vi "Initialize DAQ Instruments.vi"(8 "error in (no error)":errorcluster, 11 "DAQ":refnum<class "DAQ.lvclass">) -> (0 "error out":errorcluster, 3 "DAQ":refnum<class "DAQ.lvclass">)   [LabVIEW 2022 SP3, in "DAQ.lvclass"]
doc: "Developed by Kevin Thompson\nkevin@thompsonengineering.net\n\nCopyright 2018-2020\nThompson Engineering, LLC"
uses:
  DAQ.lvclass
  DAQ.lvclass/DAQ.ctl
  Accessors/Get DAQ Settings.vi
  Accessors/Set DI TaskNames.vi
  Accessors/Set AI TaskNames.vi
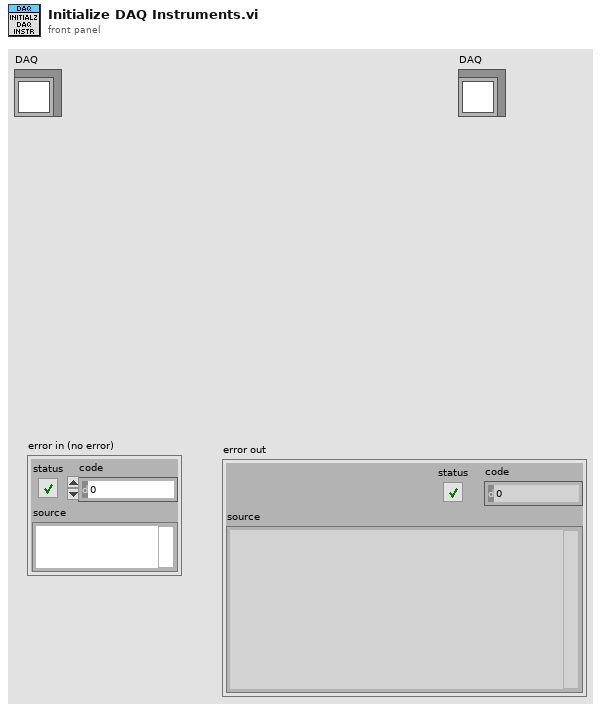
[diagram p1: front panel]
types:
  T1 = typedef "DAQ.lvclass/TD DAQ Settings--cluster.ctl" = cluster{"Simulate DAQ":bool, "DI Settings":T2[], "AI Settings":T3[], "Relay IONames":string[], "AO IONames":string[], "AO NChan SingleTask":bool}
  T2 = typedef "DAQ.lvclass/TD DI Instrument Settings--cluster.ctl" = cluster{"Disable":bool, "DI TaskName":string, "DI RefreshIntv":i32}
  T3 = typedef "DAQ.lvclass/TD AI Instrument Settings--cluster.ctl" = cluster{"Disable":bool, "AI TaskName":string, "AI InstSettings":T4, "SimAI Ranges":T5}
  T4 = typedef "DAQ.lvclass/TD AI InstSettings--cluster.ctl" = cluster{"DaqRate":dbl, "NumSamples":i32}
  T5 = typedef "DAQ.lvclass/TD SimAI Ranges--cluster.ctl" = cluster{"lo":dbl, "hi":dbl}
  T6 = typedef "TD Pathnames--cluster.ctl" = cluster{"RunTimeSys?":bool, "AppFolder":path, "ExecutablePath":path, "ConfigFolder":path, "DataLogFolder":path, "SystemLogFolder":path, "SeqFolder":path, "MainStartupPathname":path, "MainUIPathname":path, "SystemEventsFile":path, "SeqEventsFile":path, "Config SettingsFile":path, "DAQ IOConfigFile":path, "SystemSimulation":bool, "DLPUIConfigFile":path}
  T7 = typedef "TD Dynamic CVT DVR--ref.ctl" = refnum<data-value>
  T8 = typedef "DAQ.lvclass/TD IO Node Definition--cluster.ctl" = cluster{"DI Config":T9, "DO Config":T12, "AI Config":T14, "AO Config":T20}
  T9 = typedef "DAQ.lvclass/TD DI Config--cluster.ctl" = cluster{"DI Tasks":T10[]}
  T10 = typedef "DAQ.lvclass/TD DI Task--cluster.ctl" = cluster{"DI TaskName":string, "DI Channels":T11[]}
  T11 = typedef "DAQ.lvclass/TD DI Channel--cluster.ctl" = cluster{"DevName":string, "IOName":string, "IOPath":string, "SchemName":string, "logic":enum16{"Lo", "Hi"}, "Index":i32}
  T12 = typedef "DAQ.lvclass/TD DO Config--cluster.ctl" = cluster{"DO Channels":T13[]}
  T13 = typedef "DAQ.lvclass/TD DO Channel--cluster.ctl" = cluster{"DevName":string, "IOName":string, "IOPath":string, "SchemName":string, "logic":enum16{"Lo", "Hi"}, "DAQmx Task":refnum<k21>}
  T14 = typedef "DAQ.lvclass/TD AI Config--cluster.ctl" = cluster{"AI Tasks":T15[]}
  T15 = typedef "DAQ.lvclass/TD AI Task--cluster.ctl" = cluster{"AI TaskName":string, "AI Channels":T16[]}
  T16 = typedef "DAQ.lvclass/TD AI Channel--cluster.ctl" = cluster{"DevName":string, "IOName":string, "IOPath":string, "SchemName":string, "MinValue":dbl, "MaxValue":dbl, "Terminal Configuration":i32, "Index":i32, "Conversion":T17, "AIType":T18, "Force Bridge":T19}
  T17 = typedef "DAQ.lvclass/TD DataValueConversion--cluster.ctl" = cluster{"MaxSignal":dbl, "MinSignal":dbl, "MaxEngUnit":dbl, "MinEngUnit":dbl, "ScaleOffset":dbl, "negate":bool}
  T18 = typedef "DAQ.lvclass/TD AI DAQ Type--enum.ctl" = enum16{"Voltage", "Current", "Strain Gage", "Force Bridge"}
  T19 = typedef "DAQ.lvclass/TD AI Force Bridge--cluster.ctl" = cluster{"bridge information":cluster{"bridge configuration":i32, "voltage excitation source":i32, "voltage excitation value":dbl, "nominal bridge resistance":dbl}, "scaling information":cluster{"first electrical value":dbl, "second electrical value":dbl, "electrical units":i32, "first physical value":dbl, "second physical value":dbl, "physical units":i32}}
  T20 = typedef "DAQ.lvclass/TD AO Config--cluster.ctl" = cluster{"AO Channels":T21[]}
  T21 = typedef "DAQ.lvclass/TD AO Channel--cluster.ctl" = cluster{"DevName":string, "IOName":string, "IOPath":string, "SchemName":string, "Vmin":dbl, "Vmax":dbl, "Conversion":T17, "DAQmx Task":refnum<k21>}
  T22 = typedef "DAQ.lvclass/offsets cluster.ctl" = cluster{"Offset IONames":string[], "Offset Value":dbl[]}
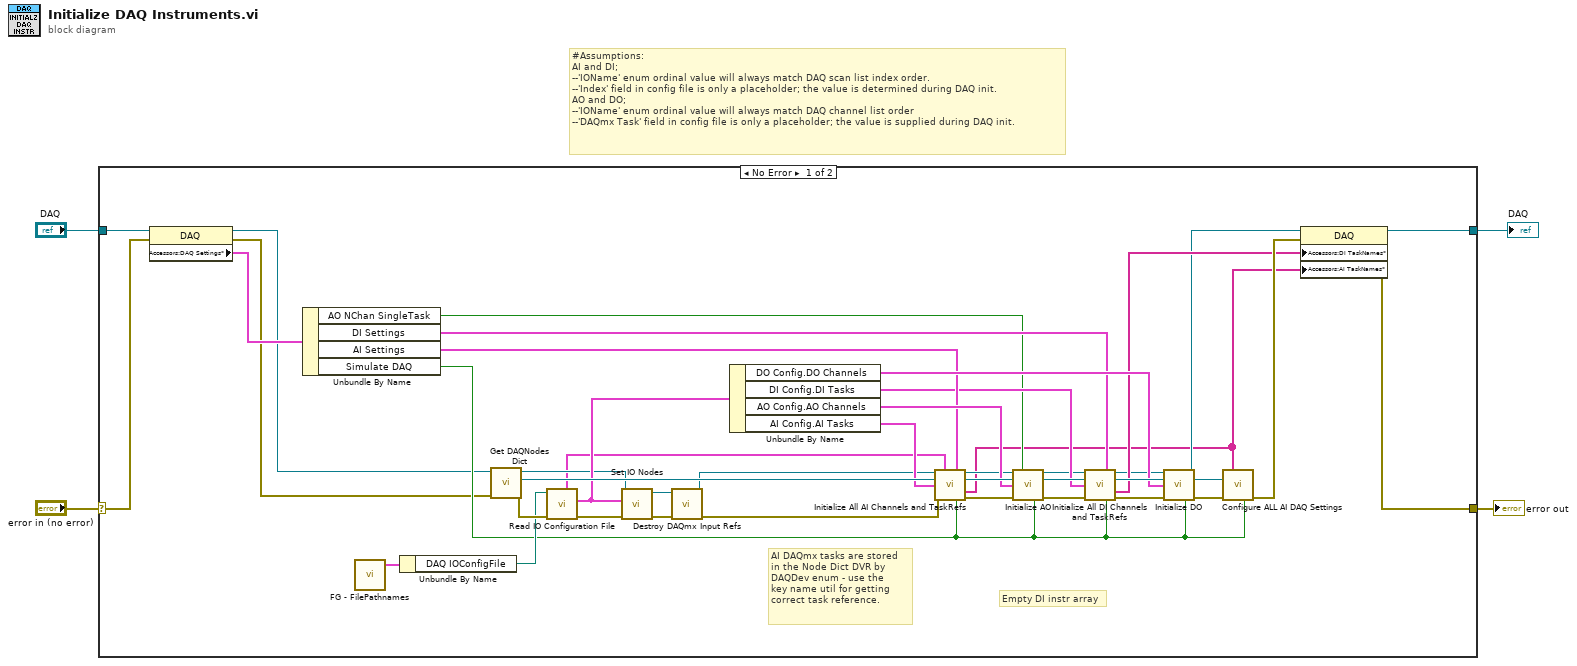
[diagram p0: block diagram]
diagram:
  # "#Assumptions:\nAI and DI;\n--'IOName' enum ordinal value will always match DAQ scan list index order.\n--'Index' field in config file is only a placeholder; the value is determined during DAQ init.\nAO and DO;\n--'IOName' enum ordinal value will always match DAQ channel list order\n--'DAQmx Task' field in config file is only a placeholder; the value is supplied during DAQ init."
  n1 = case shown="No Error" "error in (no error)" {
    selector: "error in (no error)" -> [w22 w48]
    tunnel: [w13 w48] -> w4
    tunnel: "DAQ" -> [w23 w47]
    tunnel: [w15 w47] -> w1
    frame No Error {
      # "AI DAQmx tasks are stored\nin the Node Dict DVR by\nDAQDev enum - use the\nkey name util for getting\ncorrect task reference."
      # "Empty DI instr array"
      n2 = property class="DAQ"(reference=w23, error in=w22) -> (reference out=w21:refnum<class "DAQ.lvclass">, error out=w20:errorcluster, "Accessors:DAQ Settings*"=w27:T1)
      n3 = Unbundle By Name(w27) -> ("AO NChan SingleTask"=w6:bool, "DI Settings"=w24:T2[], "AI Settings"=w30:T3[], "Simulate DAQ"=w28:bool)
      n4 = call "FG - FilePathnames.vi"() -> ("FilePaths out"=w38:T6)  [unwired: 4 in, 1 out]
      n5 = Unbundle By Name(w38) -> ("DAQ IOConfigFile"=w34:path)
      n6 = call "Get DAQNodes Dict.vi"("error in (no error)"=w20, "DAQ"=w21) -> ("error out"=w40:errorcluster, "DAQ Node Dict DVR"=w39:T7, "DAQ"=w31:refnum<class "DAQ.lvclass">)  [unwired: 7 in]
      n7 = call "Read IO Configuration File.vi"("error in (no error)"=w40, "DAQ ConfigFile"=w34) -> ("error out"=w32:errorcluster, "IO Nodes"=w33:T8, "offsets"=w19:T22)  [unwired: 5 in, 2 out]
      n8 = call "Set IO Nodes.vi"("error in (no error)"=w32, "IO Nodes"=w33, "DAQ in"=w31) -> ("error out"=w18:errorcluster, "DAQ out"=w16:refnum<class "DAQ.lvclass">)  [unwired: 7 in]
      n9 = call "Destroy DAQmx Input Refs.vi"("error in (no error)"=w18, "DAQ"=w16) -> ("error out"=w17:errorcluster, "DAQ"=w12:refnum<class "DAQ.lvclass">)  [unwired: 8 in]
      n10 = Unbundle By Name(w33) -> ("DO Config.DO Channels"=w37:T13[], "DI Config.DI Tasks"=w25:T10[], "AO Config.AO Channels"=w36:T21[], "AI Config.AI Tasks"=w26:T15[])
      n11 = call "Initialize All AI Channels and TaskRefs.vi"("DAQ"=w12, "offsets"=w19, "AI Settings[]"=w30, "DAQNode Dict"=w39, "AI Tasks"=w26, "error in"=w17, "Simulate"=w28) -> ("DAQ out"=w11:refnum<class "DAQ.lvclass">, "DAQNode Dict out"=w45:T7, "AI TaskNames"=w5:string[], "error out"=w46:errorcluster)  [unwired: 4 in, 1 out]
      n12 = call "Initialize AO.vi"("DAQ"=w11, "N Ch 1 task"=w6, "DAQNode Dict"=w45, "AO Channels"=w36, "error in"=w46, "Simulate"=w28) -> ("DAQ out"=w10:refnum<class "DAQ.lvclass">, "DAQNode Dict out"=w43:T7, "error out"=w44:errorcluster)  [unwired: 7 in]
      n13 = call "Initialize All DI Channels and TaskRefs.vi"("DAQ"=w10, "DI Settings[]"=w24, "DAQNode Dict"=w43, "DI Tasks"=w25, "error in"=w44, "Simulate"=w28) -> ("DAQ out"=w8:refnum<class "DAQ.lvclass">, "DAQNode Dict out"=w41:T7, "DI TaskNames"=w9:string[], "error out"=w42:errorcluster)  [unwired: 5 in, 1 out]
      n14 = call "Initialize DO.vi"("DAQ"=w8, "DAQNode Dict"=w41, "DO Channels"=w37, "error in"=w42, "Simulate"=w28) -> ("DAQ out"=w7:refnum<class "DAQ.lvclass">, "DAQNode Dict out"=w29:T7, "error out"=w35:errorcluster)  [unwired: 8 in]
      n15 = call "Configure ALL AI DAQ Settings.vi"("AI TaskNames"=w5, "DAQNode Dict"=w29, "error in (no error)"=w35, "Simulate"=w28) -> ("error out"=w14:errorcluster)  [unwired: 10 in, 1 out]
      n16 = property class="DAQ"(reference=w7, error in=w14, "Accessors:DI TaskNames*"=w9, "Accessors:AI TaskNames*"=w5) -> (reference out=w15:refnum<class "DAQ.lvclass">, error out=w13:errorcluster)
    }
    frame Error {
    }
  }
  "error out" <- w4
  "DAQ" <- w1
